vi "Update PDO Count.vi"(8 "error in":errorcluster, 11 "EDS in":refnum<class "Electronic Datasheet.lvclass">) -> (0 "error out":errorcluster, 3 "EDS out":refnum<class "Electronic Datasheet.lvclass">)   [LabVIEW 2019, in "Electronic Datasheet.lvlib" / "Electronic Datasheet.lvclass"]
uses:
  Electronic Datasheet.lvclass
  Electronic Datasheet.lvclass/Electronic Datasheet.ctl
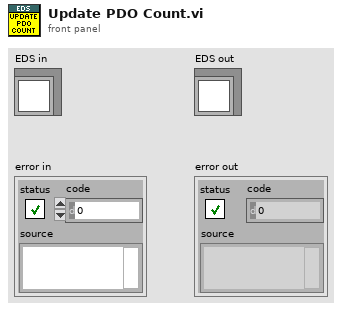
[diagram p1: front panel]
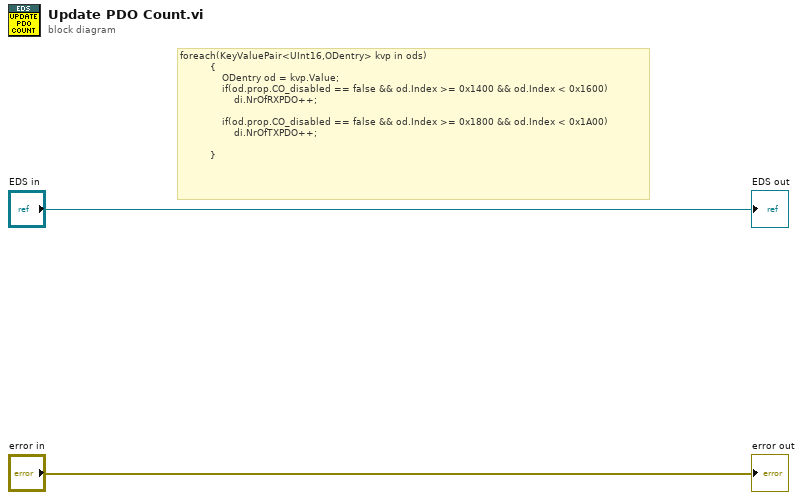
[diagram p0: block diagram]
diagram:
  # "foreach(KeyValuePair<UInt16,ODentry> kvp in ods)\n          {\n              ODentry od = kvp.Value;\n              if(od.prop.CO_disabled == false && od.Index >= 0x1400 && od.Index < 0x1600)\n                  di.NrOfRXPDO++;\n\n              if(od.prop.CO_disabled == false && od.Index >= 0x1800 && od.Index < 0x1A00)\n                  di.NrOfTXPDO++;\n\n          }"
  "error out" <- "error in"
  "EDS out" <- "EDS in"
